vi "HTS_INJECTION_LIST.vi"(8 "Error IN":errorcluster, 10 "Wells  to inject (Well array)":T1[](array[typedef])) -> (0 "Error OUT":errorcluster, 2 "Commands (String Array)":string[](array[string]))   [LabVIEW 2009]
uses:
  HTS_WELL.ctl
  HTS_COLUMN.ctl
  HTS_ROW.ctl
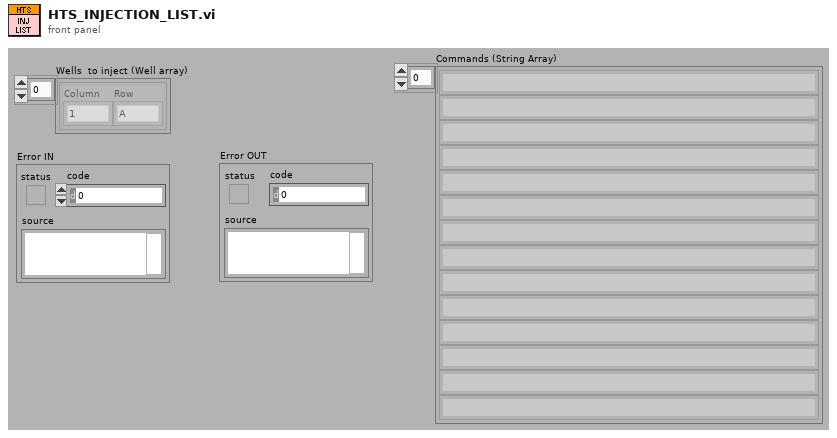
[diagram p1: front panel]
types:
  T1 = typedef "HTS_WELL.ctl" = cluster{"Column":T2, "Row":T3}
  T2 = typedef "HTS_COLUMN.ctl" = enum16{"1", "2", "3", "4", "5", "6", "7", "8", "9", "10", "11", "12"}
  T3 = typedef "HTS_ROW.ctl" = enum16{"A", "B", "C", "D", "E", "F", "G", "H"}
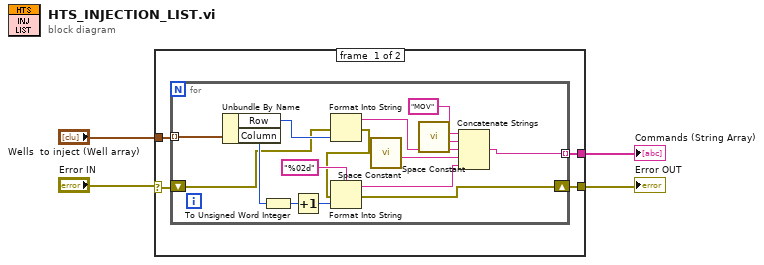
[diagram p0: block diagram]
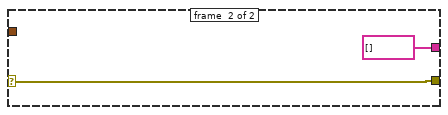
[diagram p2: hidden frame]
diagram:
  n1 = case shown="No Error" "Error IN" {
    selector: "Error IN" -> [w5 w25]
    tunnel: "Wells  to inject (Well array)" -> [w8 _]
    tunnel: [w7 string[] []] -> w3
    tunnel: [w6 w25] -> w2
    frame #0 {
      n2 = for {
        tunnel: w8 -> [w23] mode=indexing
        tunnel: [w19] -> w7 mode=indexing
        shift-right: [w10] -> w6
        shift-left: w5 -> [w9]
        n3 = Unbundle By Name(w23) -> ("Row"=w22:T3, "Column"=w18:T2)
        n4 = To Unsigned Word Integer(number=w18) -> (unsigned 16bit integer=w14:u16)
        n5 = Increment(x=w14) -> (x+1=w15:u16)
        n6 = Format Into String(error in=w9, w22) -> (resulting string=w20:string, error out=w11:errorcluster)  [unwired: 2 in]
        n7 = Format Into String(format string="%02d", error in=w11, w15) -> (resulting string=w16:string, error out=w10:errorcluster)  [unwired: 1 in]
        n8 = call <vilib>:"Space Constant.vi"() -> ("String"=w21:string)
        n9 = call <vilib>:"Space Constant.vi"() -> ("String"=w13:string)
        n10 = Concatenate Strings("MOV" ("string"), w13, w20, w21, w16) -> (w19:string)
      }
    }
    frame #1 {
    }
  }
  "Commands (String Array)" <- w3
  "Error OUT" <- w2
